vi "LaunchVeriStand.vi"(8 "error in (no error)":errorcluster) -> (0 "error out":errorcluster)   [LabVIEW 2015, in "VeriStandTestCase.lvclass"]
uses:
  VeriStandTestCase.lvclass
  <vilib>/Utility/sysdir.llb/System Directory Type.ctl
panel:
  out "Command to launch VS":string
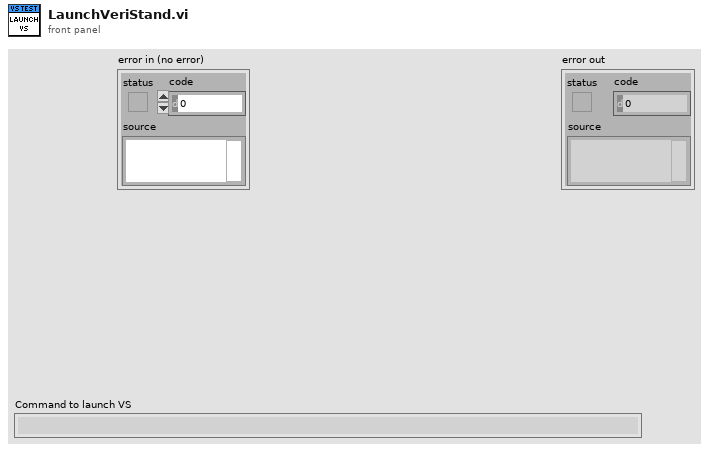
[diagram p1: front panel]
types:
  T1 = typedef "System Directory Type.ctl" = i32
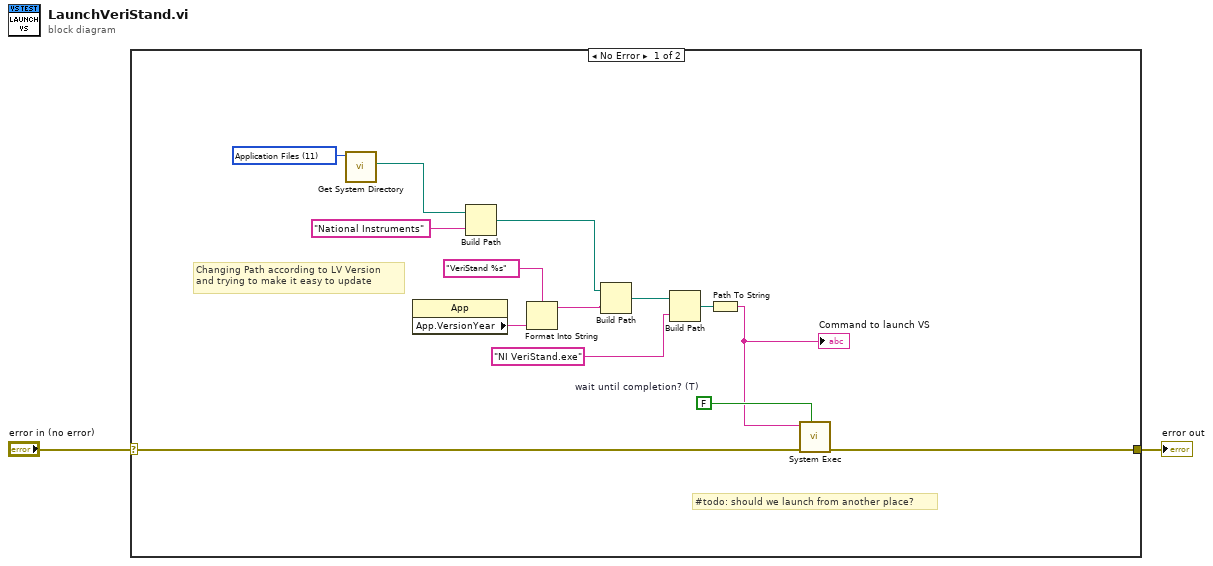
[diagram p0: block diagram]
diagram:
  n1 = case shown="No Error" "error in (no error)" {
    selector: "error in (no error)" -> [w5 w17]
    tunnel: [w3 w17] -> w1
    frame No Error {
      w14 = T1 11 items=["User Home"=0, "User Desktop"=1, "User Documents"=2, "User Application Data"=3, "User Preferences"=4, "User Temporary"=5, "Public Documents"=6, "Public Application Data"=7, "Public Preferences"=8, "Public Cache"=13, "System Core Libraries"=9, "System Installed Libraries"=10, "Application Files"=11, "Boot Volume Root"=12] ("system directory type")
      w16 = FALSE  # wait until completion? (T)
      # "Changing Path according to LV Version\nand trying to make it easy to update"
      # "#todo: should we launch from another place?"
      n2 = call <vilib>:"Get System Directory.vi"("system directory type"=w14) -> ("system directory"=w12:path)  [unwired: 10 in]
      n3 = property class="App"() -> ("App.VersionYear"=w15:string)  [unwired: 2 in, 2 out]
      n4 = Build Path(base path=w12, name or relative path="National Instruments" ("command line")) -> (appended path=w11:path)
      n5 = Format Into String(format string="VeriStand %s" ("command line"), w15) -> (resulting string=w10:string)  [unwired: 2 in, 1 out]
      n6 = Build Path(base path=w11, name or relative path=w10) -> (appended path=w7:path)
      n7 = Build Path(base path=w7, name or relative path="NI VeriStand.exe" ("command line")) -> (appended path=w6:path)
      n8 = Path To String(path=w6) -> (string=w9:string)
      "Command to launch VS" <- w9
      n9 = call <vilib>:"System Exec.vi"("wait until completion? (T)"=w16, "error in (no error)"=w5, "command line"=w9) -> ("error out"=w3:errorcluster)  [unwired: 5 in, 3 out]
    }
    frame Error {
    }
  }
  "error out" <- w1
